vi "FastLocalizeCPU.vi"(0 "tracker":u64, 2 "input image":T1, 3 "debug image":T1) -> (6 "tracker":u64, 7 "COM":cluster{"comX":sgl, "comY":sgl}, 8 "debug image":T1(plugin-control), 9 "xcorpos":cluster{"XCor X":sgl, "XCor Y":sgl}, 10 "median":sgl)   [LabVIEW 2011]
uses:
  <vilib>/vision/Image Controls.llb/IMAQ Image.ctl
  CpuTrackDLL.vi
panel:
  in  "XCor X":sgl
  in  "XCor Y":sgl
  in  "comX":sgl
  in  "comY":sgl
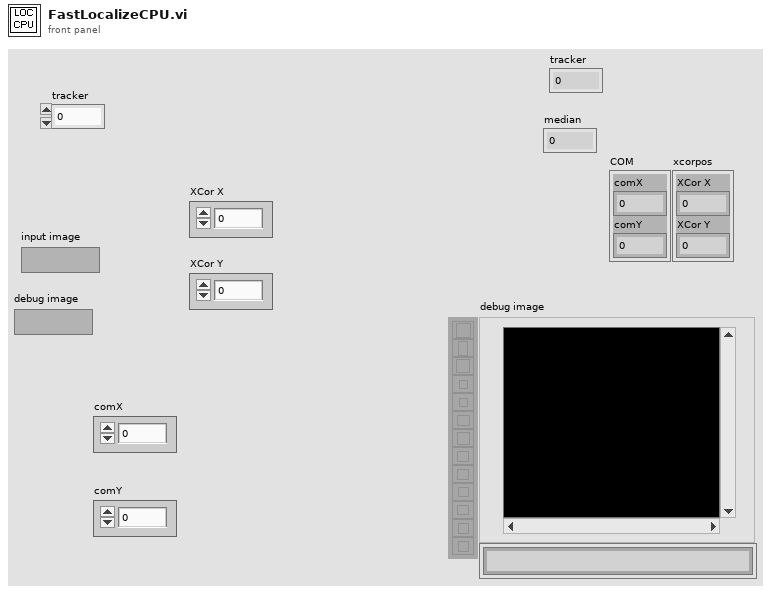
[diagram p1: front panel]
types:
  T1 = typedef "IMAQ Image.ctl" = refnum<image>
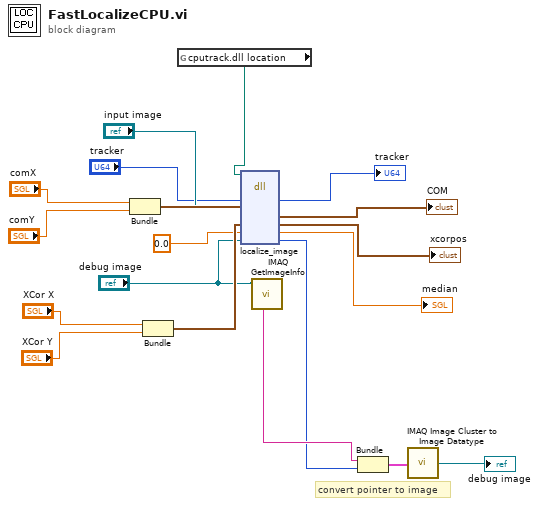
[diagram p0: block diagram]
diagram:
  # "convert pointer to image"
  n1 = Bundle("comX"="comX", "comY"="comY") -> (w17:cluster{"comX":sgl, "comY":sgl})  [unwired: 1 in]
  n2 = Bundle("XCor X"="XCor X", "XCor Y"="XCor Y") -> (w14:cluster{"XCor X":sgl, "XCor Y":sgl})  [unwired: 1 in]
  n3 = global read "CpuTrackDLL.vi" "cputrack.dll location"() -> (w3:path)
  n4 = dll-call lib="D:/jcnossen1/cudaqi-tracker/Debug/cputrack.dll" fn="localize_image"(path in=w3, "tracker"="tracker", "image"="input image", "COM"=w17, "xcorpos"=w14, "median"=sgl 0.0, "debugImage"="debug image") -> ("tracker"=→"tracker":u64, "COM"=→"COM":cluster{"comX":sgl, "comY":sgl}, "xcorpos"=→"xcorpos":cluster{"XCor X":sgl, "XCor Y":sgl}, "median"=→"median":sgl, "debugImage"=w4:u64)  [unwired: 4 in, 2 out]
  n5 = call "IMAQ GetImageInfo"("Image"="debug image") -> ("Image Name"=w6:string)  [unwired: 3 in, 7 out]
  n6 = Bundle("Image Name"=w6, "debugImage"=w4) -> (w7:cluster{"Image Name":string, "debugImage":u64})  [unwired: 1 in]
  n7 = call <vilib>:"IMAQ Image Cluster to Image Datatype.vi"("Image"=w7) -> ("Image (dup)"=→"debug image":T1)
